vi "Calibrate photo-stimulation.vi"() -> ()   [LabVIEW 2017]
panel:
  in  "Light ON":bool
  in  "stop":bool
  in  "Calibration data (update values manually!)":string
  out "Output voltage":dbl
  in  "Max output voltage":dbl min=0.0 max=5.0
  in  "Min output voltage (threshold current)":dbl min=0.0 max=5.0
  in  "Stimulus range":dbl(slide)=1.0 min=0.0 max=1.0 step=0.05 scale=0.0..1.0
  # "Mapping Command voptage to light output \n\nCalibration step by step: \n\n1) Measure the diameter of the stimulus light at the focal plane of the sample and calculate the required total light intensity. \n\n2) Find the required light output by adjusting the \"Max voltage output\" \n\n3) Find the command voltage corresponds to the threshold current of the laser diode by adjusting the \"Max output voltage \" or the \"Stimulus range slider\".  This value is the lower end of the linear scale\n\n4) Optional: update the \"Min output voltage\" value based on the previous step. When both the Min and Max output voltage are correct the \"Stimulus range\" slider should represent the linear range that will be available in the experimental VI.\n\n5) Update all the measured values in the text editor window. The data is saved in a text file and will be read by the experimental VI (VR controller) therefore it is important that it contains the data in the text format below. The entire \"Calibration data\" text will be added to the labbook file of the experiments.\n\n\n\nDescription have to contain:\n\n\"Min output: #.# V, light intensity: #.# mW\nMax output: #.# V, light intensity: #.# mW\""
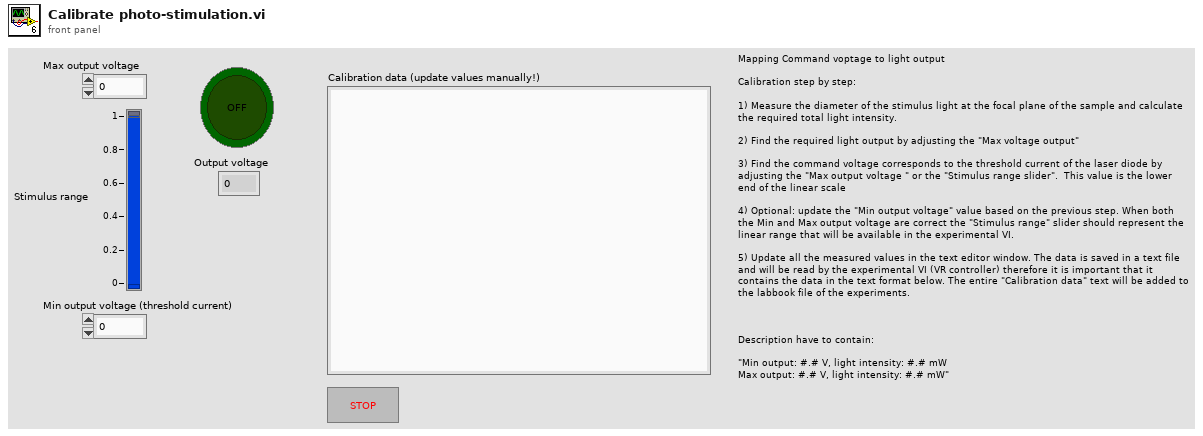
[diagram p1: front panel]
types:
  T1 = enum16{"open", "replace", "create", "open or create", "replace or create", "replace or create with confirmation"}
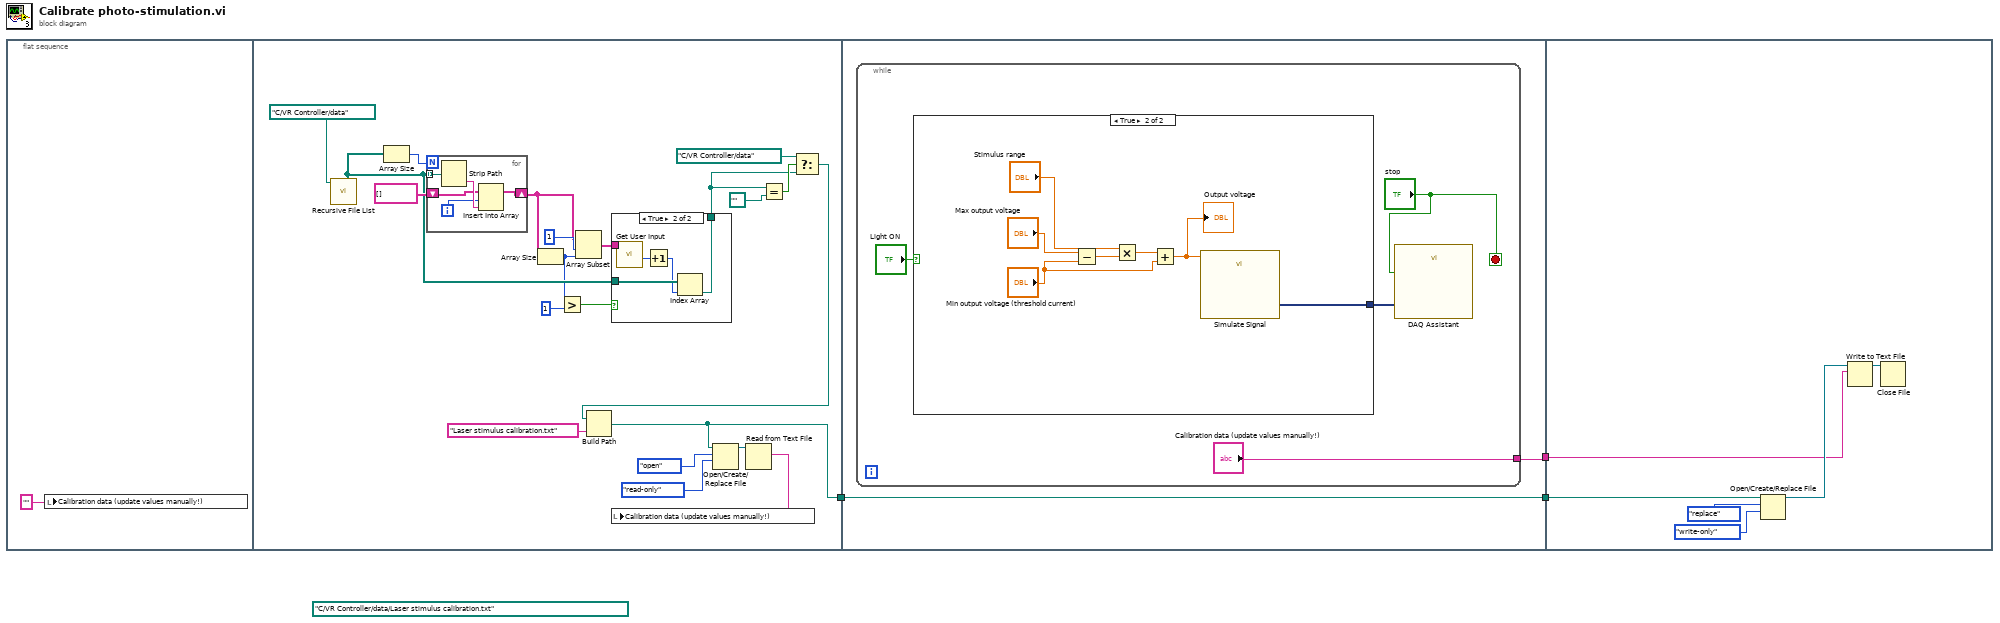
[diagram p0: block diagram]
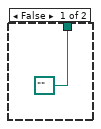
[diagram p2: hidden frame]
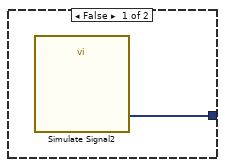
[diagram p3: hidden frame]
diagram:
  (unwired) path "C:/VR Controller/data/Laser stimulus calibration.txt" ("file path (dialog if empty)")
  n1 = flat-sequence {
    tunnel: [w5] -> w1
    tunnel: [w38] -> w3
    tunnel: [w37] -> w2
    tunnel: w1 -> [w37]
    tunnel: w3 -> [w51]
    tunnel: w2 -> [w52]
    frame #0 {
      n2 = local write "Calibration data (update values manually!)"("" ("Calibration data (update values manually)")) -> ()
    }
    frame #1 {
      n3 = call <vilib>:"Recursive File List.vi"("Folder Path"=path "C:/VR Controller/data" ("path")) -> ("All Folders"=w16:path[])  [unwired: 6 in, 4 out]
      n4 = Array Size(array=w16) -> (size(s)=w21:i32)
      n5 = for {
        N: w21 -> [_]
        tunnel: w16 -> [w36] mode=indexing
        shift-right: [w33] -> w18
        shift-left: string[] [] -> [w32]
        i -> [w34]
        n6 = Strip Path(path=w36) -> (name=w35:string)  [unwired: 1 out]
        n7 = Insert Into Array(array=w32, index=w34, new element=w35) -> (w33:string[])
      }
      n8 = Array Size(array=w18) -> (size(s)=w10:i32)
      n9 = Greater?(x=w10, y=1) -> (0:w8:bool)
      n10 = Array Subset(array=w18, index=1, length=w10) -> (w17:string[])
      n11 = case shown="True" w8 {
        tunnel: w17 -> [_ w31]
        tunnel: w16 -> [_ w30]
        tunnel: [path "" ("path") w27] -> w12
        frame False {
        }
        frame True {
          n12 = call "Get User Input.vi"("Strings []"=w31) -> ("user"=w29:u16)  [unwired: 1 in, 9 out]
          n13 = Increment(x=w29) -> (x+1=w28:u16)
          n14 = Index Array(array=w30, index=w28) -> (element=w27:path)
        }
      }
      n15 = Equal?(x=w12, y=path "" ("path")) -> (x = y?=w14:bool)
      n16 = Select(t=path "C:/VR Controller/data", s=w14, f=w12) -> (s? t:f=w6:path)
      n17 = Build Path(base path=w6, name or relative path="Laser stimulus calibration.txt") -> (appended path=w5:path)
      n18 = Open/Create/Replace File(file path (use dialog)=w5, operation (0:open)=T1."open", access (0:read/write)=enum16{"read/write", "read-only", "write-only"}."read-only") -> (refnum out=w24:refnum<file>)  [unwired: 3 in, 2 out]
      n19 = Read from Text File(file (use dialog)=w24) -> (text=w23:string)  [unwired: 3 in, 3 out]
      n20 = local write "Calibration data (update values manually!)"(w23) -> ()
    }
    frame #2 {
      n21 = while {
        tunnel: ["Calibration data (update values manually!)"] -> w38
        stop <- "stop" stop-if-true
        n22 = case shown="True" "Light ON" {
          tunnel: [w43 w44] -> w42
          frame False {
            n23 = call "Simulate Signal2"() -> ("DC"=w43:dynamicdata)  [unwired: 14 in, 1 out]
          }
          frame True {
            n24 = Subtract(x="Max output voltage", y="Min output voltage (threshold current)") -> (x-y=w48:dbl)
            n25 = Multiply(x="Stimulus range", y=w48) -> (x*y=w49:dbl)
            n26 = Add(x=w49, y="Min output voltage (threshold current)") -> (x+y=w45:dbl)
            "Output voltage" <- w45
            n27 = call "Simulate Signal"("Offset"=w45) -> ("DC"=w44:dynamicdata)  [unwired: 13 in, 1 out]
          }
        }
        n28 = call "DAQ Assistant"("data"=w42, "stop (T)"="stop") -> ()  [unwired: 16 in, 2 out]
      }
    }
    frame #3 {
      n29 = Open/Create/Replace File(file path (use dialog)=w52, operation (0:open)=T1."replace", access (0:read/write)=enum16{"read/write", "read-only", "write-only"}."write-only") -> (refnum out=w56:refnum<file>)  [unwired: 3 in, 2 out]
      n30 = Write to Text File(file (use dialog)=w56, text=w51) -> (refnum out=w55:refnum<file>)  [unwired: 2 in, 2 out]
      n31 = Close File(refnum=w55) -> ()  [unwired: 1 in, 2 out]
    }
  }
